vi "Check_Control_Conflicts.vi"(8 "error in (no error)":errorcluster, 10 "Master Device in":refnum<class "Master Device.lvclass">, 11 "Device in":refnum<class "Master Device.lvclass">) -> (0 "error out":errorcluster, 1 "Controlled Channels":bool[](array[boolean]), 2 "Master Device out":refnum<class "Master Device.lvclass">, 3 "Device out":refnum<class "Master Device.lvclass">)   [LabVIEW 2013, in "Master Device.lvclass"]
uses:
  Master Device.lvclass
  Master Device.lvclass/Master Device.ctl
  <vilib>/Utility/error.llb/DialogType.ctl
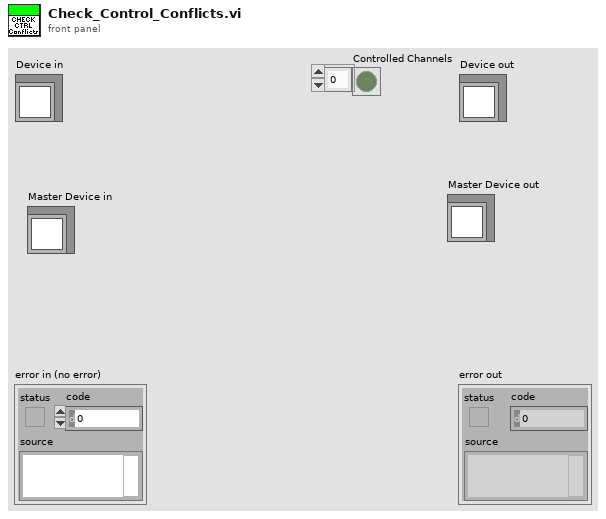
[diagram p1: front panel]
types:
  T1 = cluster{"Master Channel Number":i32, "Output States":bool[]}[]
  T2 = typedef "DialogType.ctl" = u16
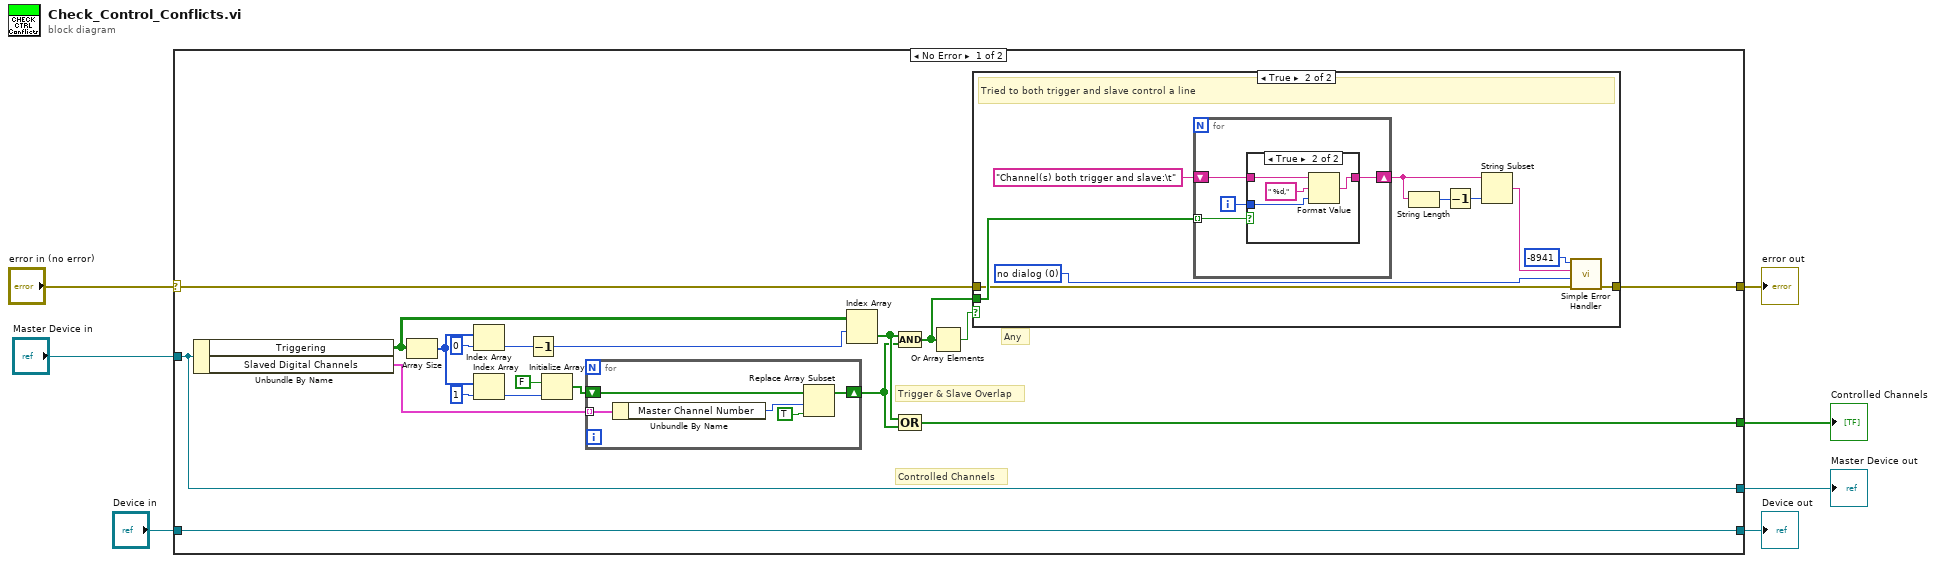
[diagram p0: block diagram]
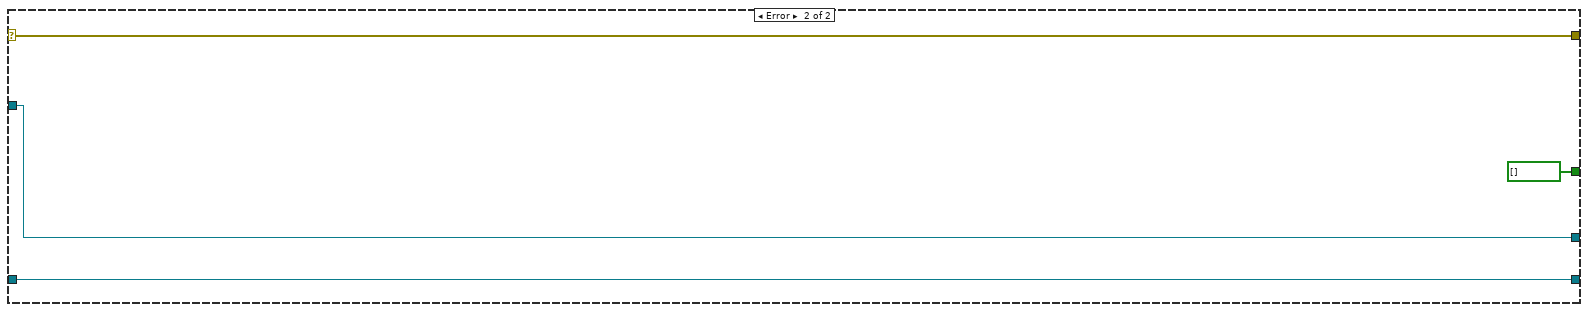
[diagram p4: hidden frame]
diagram:
  n1 = case shown="No Error" "error in (no error)" {
    selector: "error in (no error)" -> [w10 w55]
    tunnel: [w9 w55] -> w5
    tunnel: [w12 w54] -> w1
    tunnel: "Device in" -> [w12 w54]
    tunnel: "Master Device in" -> [w11 w53]
    tunnel: [w11 w53] -> w2
    tunnel: [w8 bool[] []] -> w3
    frame No Error {
      # "Controlled Channels"
      # "Trigger & Slave Overlap"
      # "Any"
      n2 = Unbundle By Name(w11) -> ("Triggering"=w26:bool[][], "Slaved Digital Channels"=w24:T1)
      n3 = Array Size(array=w26) -> (size(s)=w15:i32[])
      n4 = Index Array(array=w15, index=0) -> (element=w23:i32)
      n5 = Index Array(array=w15, index=1) -> (element=w13:i32)
      n6 = Decrement(x=w23) -> (x-1=w16:i32)
      n7 = Initialize Array(FALSE, w13) -> (w21:bool[])
      n8 = for {
        shift-right: [w49] -> w19
        shift-left: w21 -> [w51]
        tunnel: w24 -> [w48] mode=indexing
        n9 = Unbundle By Name(w48) -> ("Master Channel Number"=w47:i32)
        n10 = Replace Array Subset(array=w51, new element=TRUE, index=w47) -> (w49:bool[])
      }
      n11 = Index Array(array=w26, index (row)=w16) -> (element=w20:bool[])  [unwired: 1 in]
      n12 = Compound Arithmetic op=AND(w20, w19) -> (w17:bool[])
      n13 = Compound Arithmetic op=OR(w20, w19) -> (w8:bool[])
      n14 = Or Array Elements(Boolean array=w17) -> (logical OR=w18:bool)
      n15 = case shown="True" w18 {
        tunnel: w10 -> [w27 w32]
        tunnel: w17 -> [_ w37]
        tunnel: [w27 w28] -> w9
        frame False {
          # "No problems"
        }
        frame True {
          w30 = T2 0 items=["no dialog", "OK message", "continue or stop message", "OK message + warnings", "continue/stop + warnings"] ("type of dialog (OK msg:1)")
          # "Tried to both trigger and slave control a line"
          n16 = for {
            tunnel: w37 -> [w41] mode=indexing
            shift-right: [w39] -> w35
            shift-left: "Channel(s) both trigger and slave:\t" -> [w40]
            i -> [w38]
            n17 = case shown="True" w41 {
              tunnel: w40 -> [w42 w46]
              tunnel: [w42 w43] -> w39
              tunnel: w38 -> [_ w44]
              frame False {
              }
              frame True {
                n18 = Format Value(string ("")=w46, format string=" %d,", value (0)=w44) -> (output string=w43:string)
              }
            }
          }
          n19 = String Length(string=w35) -> (length=w34:i32)
          n20 = Decrement(x=w34) -> (x-1=w33:i32)
          n21 = String Subset(string=w35, length (rest)=w33) -> (substring=w31:string)  [unwired: 1 in]
          n22 = call <vilib>:"Simple Error Handler.vi"("error code (no error:0)"=-8941, "error source (\" \")"=w31, "type of dialog (OK msg:1)"=w30, "error in (no error)"=w32) -> ("error out"=w28:errorcluster)  [unwired: 1 in, 4 out]
        }
      }
    }
    frame Error {
    }
  }
  "error out" <- w5
  "Device out" <- w1
  "Master Device out" <- w2
  "Controlled Channels" <- w3
